vi "single sweep - save rus data.vi"(6 "channel name(s) in (Untitled)":string[](array[string])=["Frequency", "Signal_X", "Signal_Y", "IF_X", "IF_Y"], 7 "save freq units":enum16{"kHz", "Hz"}(ring), 8 "error in (no error)":errorcluster, 9 "rus response":cdb[](array[numeric]), 10 "F Array":dbl[](array[numeric]), 11 "RUS settings":T1={"NI-DAQ lockin settings"={"Samples per sine wave"=0, "Sine waves per freq step"=0, "Output Representation"=enum."Real/Imaginary", "Low-pass filter"=enum."Butterworth", "Ranges and couplings "=[]}, "Fast swep settings"={"Update rate (Hz)"=250.0, "Start F, Hz"=200000.0, "Stop F"=1700000.0, "Number of points"=30000, "Amplitude"=2.1, "Init&amplitude"=TRUE, "IF"=1000.0, "Time constant"=0.1}, "Pre-sweep delay, s"=0.0, "Lockin mode"=enum."NI-DAQ", "SR Lockin"="GPIB0::10::INSTR", "DAQmx Device"="Dev3", "Clock Multiplier"=64, "Fast Sweep Data Out"={"DO clock task"="", "DO task"="", "Update clock task"="", "DAQ lockin task"="", "Pre-sweep counter task"=""}, "Lockin Range, V"=0.0, "F Array"=[], "Freq. update clock terminal"="", "DO Clock Rate (Hz)"=5000000.0, "ADC clock terminal"="/PFI4", "Pre-sweep counter terminal"="", "Samples per read"=10, "DO clock terminal"="", "Pre-sweep points"=0, "F points per write"=1000, "Total sweep time, s"=0.0, "Initial SYNTH phase"=0.0, "Record IF"=FALSE, "Save data settings"={"Save data"=TRUE, "Data Root Path"=path "", "File Prefix"="", "File Format"=enum."ASCII", "Save column names"=TRUE, "File Comments"="<Description of the current file>", "User/Prj"="<User Name/Project Description>"}, "Data file path"=path "", "New data user event"=refnum, "Stop user event"=refnum, "Number of channels"=1, "Auto-phase"=FALSE, "RP Transeiver"=refnum} {"Lockin Range, V" format="%#_6e"; "Fast swep settings"."IF" format="%#_6p"; "Fast swep settings"."Amplitude" min=0.0 max=2.5; "Fast swep settings"."Number of points" format="%.0p"; "Fast swep settings"."Stop F" format="%#_6p"; "Fast swep settings"."Start F, Hz" format="%#_6p"; "Fast swep settings"."Update rate (Hz)" format="%0.2f"; "NI-DAQ lockin settings"."Ranges and couplings"."Coupling" items=["default"=-1, "RSE"=10083, "NRSE"=10078, "Differential"=10106, "Pseudodifferential"=12529]}) -> (0 "error out":errorcluster, 3 "Actual file path":path=path "C:/data/RUS/RUS-YBCO-Jan2011/Sample2/Round2/singlesweep/March_2011/030111/280.36300K_1500_2500_008_030111.dat")   [LabVIEW 2016]
uses:
  resonant_ultrasound/Libraries/RUS/Controls/RUS settings.ctl
  NHMFL_Core/Libraries/Red Pitaya/RP Core/RP Transceiver/RP Transceiver.lvclass
  resonant_ultrasound/Libraries/RUS/Controls/RUS NI-DAQ Lockin Settings.ctl
  resonant_ultrasound/Libraries/RUS/Controls/Sweep settings.ctl
  resonant_ultrasound/Libraries/RUS/Controls/Lockin mode.ctl
  NHMFL_Core/Libraries/File/Controls/Save data settings.ctl
  NHMFL_Core/Libraries/File/Controls/File formats.ctl
  NHMFL_Core/Libraries/File/Save Data DBL.vi
panel:
  in  "Signal":dbl[][](array[numeric])
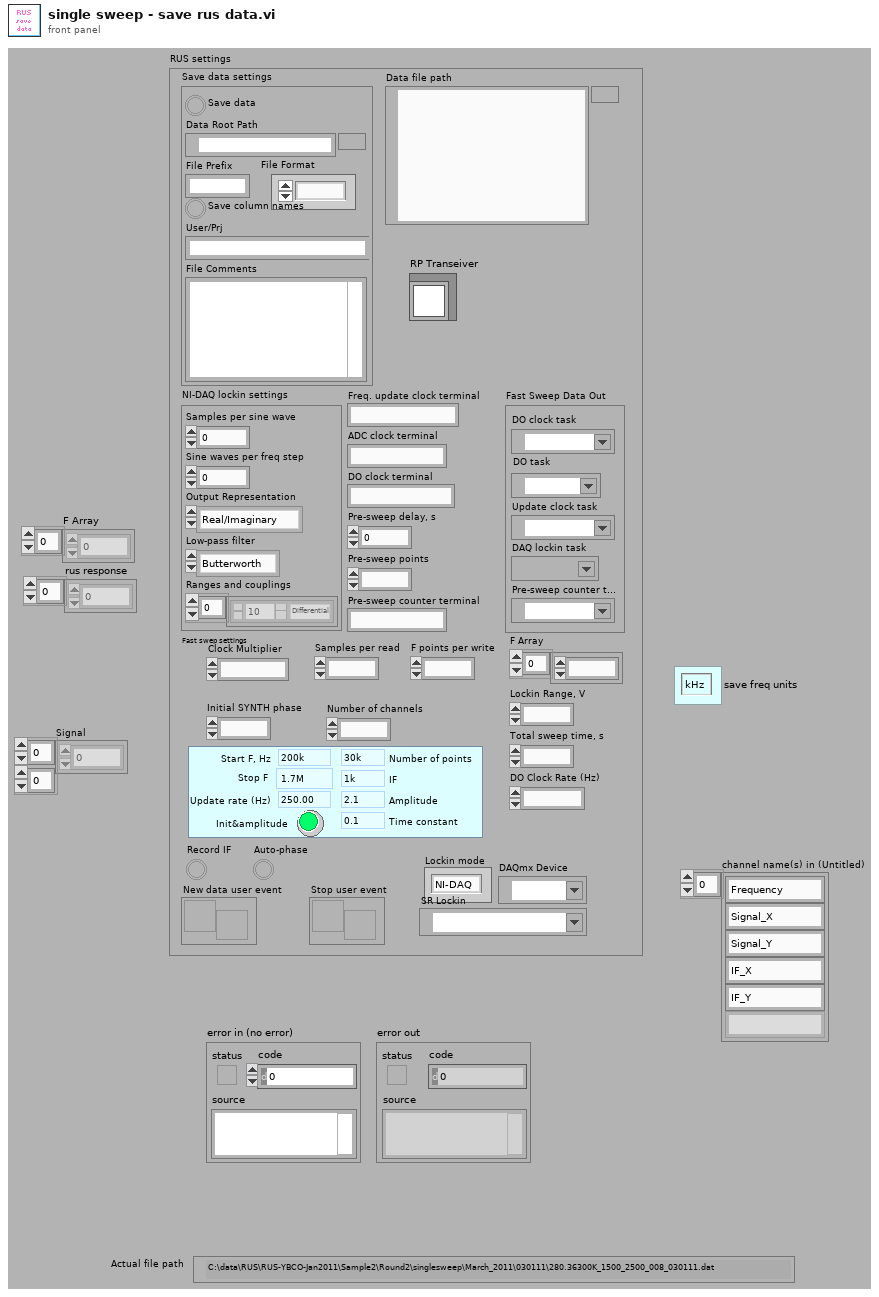
[diagram p1: front panel]
types:
  T1 = typedef "RUS settings.ctl" = cluster{"NI-DAQ lockin settings":T2, "Fast swep settings":T3, "Pre-sweep delay, s":dbl, "Lockin mode":T4, "SR Lockin":refnum<visa-resource-name>, "DAQmx Device":tag, "Clock Multiplier":i32, "Fast Sweep Data Out":cluster{"DO clock task":refnum<k21>, "DO task":refnum<k21>, "Update clock task":refnum<k21>, "DAQ lockin task":refnum<k21>, "Pre-sweep counter task":refnum<k21>}, "Lockin Range, V":sgl, "F Array":dbl[], "Freq. update clock terminal":string, "DO Clock Rate (Hz)":dbl, "ADC clock terminal":string, "Pre-sweep counter terminal":string, "Samples per read":i32, "DO clock terminal":string, "Pre-sweep points":i32, "F points per write":i32, "Total sweep time, s":dbl, "Initial SYNTH phase":dbl, "Record IF":bool, "Save data settings":T5, "Data file path":path, "New data user event":refnum<user-event>, "Stop user event":refnum<user-event>, "Number of channels":i32, "Auto-phase":bool, "RP Transeiver":refnum<class "RP Transceiver.lvclass">}
  T2 = typedef "RUS NI-DAQ Lockin Settings.ctl" = cluster{"Samples per sine wave":i32, "Sine waves per freq step":i32, "Output Representation":enum16{"Real/Imaginary", "Polar"}, "Low-pass filter":enum16{"No filtering", "Butterworth", "Bessel"}, "Ranges and couplings ":cluster{"Range":dbl, "Coupling":i32}[]}
  T3 = typedef "Sweep settings.ctl" = cluster{"Update rate (Hz)":dbl, "Start F, Hz":dbl, "Stop F":dbl, "Number of points":i32, "Amplitude":dbl, "Init&amplitude":bool, "IF":dbl, "Time constant":dbl}
  T4 = typedef "Lockin mode.ctl" = enum16{"SRS", "NI-DAQ", "Pitaya"}
  T5 = typedef "Save data settings.ctl" = cluster{"Save data":bool, "Data Root Path":path, "File Prefix":string, "File Format":T6, "Save column names":bool, "File Comments":string, "User/Prj":string}
  T6 = typedef "File formats.ctl" = enum16{"TDMS", "ASCII", "BINARY"}
  T7 = cluster{"Data file path":path, path, "channel name(s) in (Untitled)":string[]}
  T8 = typedef "Save data details.ctl" = cluster{"Data file path":path, "Comments file path":path, "Channel names":string[]}
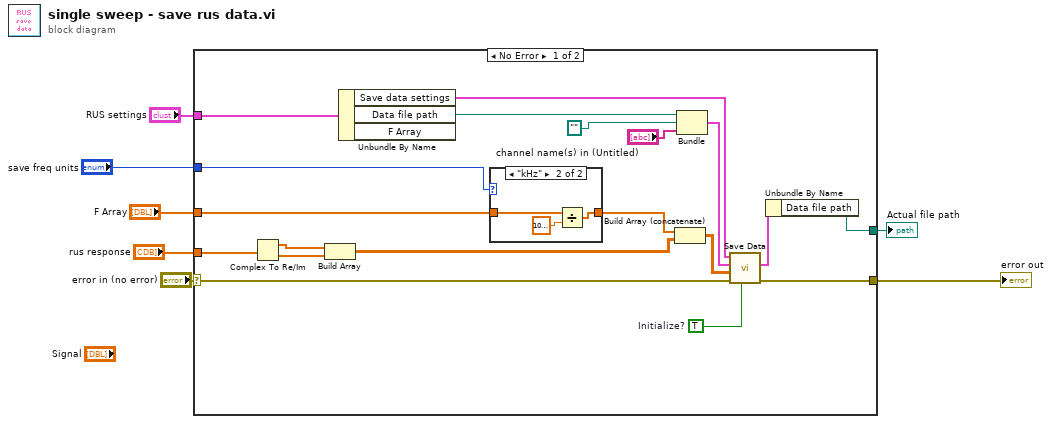
[diagram p0: block diagram]
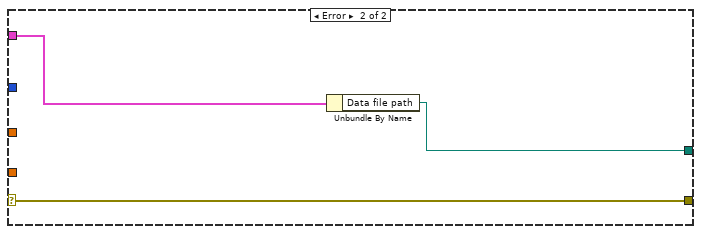
[diagram p3: hidden frame]
diagram:
  n1 = case shown="No Error" "error in (no error)" {
    selector: "error in (no error)" -> [w16 w31]
    tunnel: [w19 w32] -> w7
    tunnel: [w18 w31] -> w6
    tunnel: "RUS settings" -> [w15 w33]
    tunnel: "rus response" -> [w10 _]
    tunnel: "F Array" -> [w9 _]
    tunnel: "save freq units" -> [w8 _]
    frame No Error {
      w17 = TRUE  # Initialize?
      n2 = Complex To Re/Im(x + iy=w10) -> (x=w14:dbl[], y=w13:dbl[])
      n3 = Build Array(w14, w13) -> (w11:dbl[][])
      n4 = Unbundle By Name(w15) -> ("Save data settings"=w25:T5, "Data file path"=w24:path)  [unwired: 1 out]
      n5 = case shown="\"kHz\"" w8 {
        tunnel: [w27 w29] -> w26
        tunnel: w9 -> [w27 w28]
        frame "Hz", Default {
        }
        frame "kHz" {
          n6 = Divide(x=w28, y=1000.0) -> (x/y=w29:dbl[])
        }
      }
      n7 = Build Array (concatenate)(w26, w11) -> (w12:dbl[][])
      n8 = Bundle("Data file path"=w24, path "", "channel name(s) in (Untitled)"="channel name(s) in (Untitled)") -> (w21:T7)  [unwired: 1 in]
      n9 = call-poly "Save Data.vi"("Initialize?"=w17, "error in (no error)"=w16, "Data"=w12, "Save data details"=w21, "Save data settings"=w25) -> ("error out"=w18:errorcluster, "Save data details out"=w20:T8)  [unwired: 5 in]
      n10 = Unbundle By Name(w20) -> ("Data file path"=w19:path)
    }
    frame Error {
      n11 = Unbundle By Name(w33) -> ("Data file path"=w32:path)
    }
  }
  "Actual file path" <- w7
  "error out" <- w6
